vi "Unbox.vi"(10 "CustomeData in":refnum<class "CustomeData.lvclass">) -> (2 "data":i32)   [LabVIEW 2010, in "CustomeData.lvclass"]
uses:
  CustomeData.lvclass
  CustomeData.lvclass/CustomeData.ctl
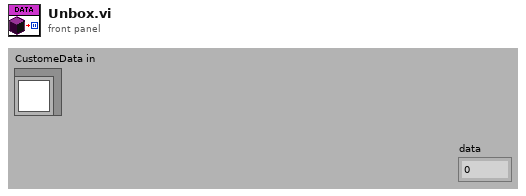
[diagram p1: front panel]
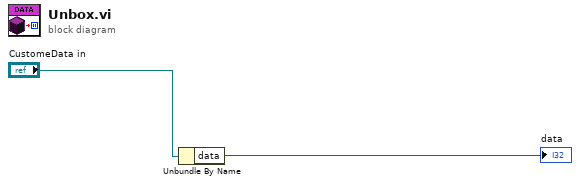
[diagram p0: block diagram]
diagram:
  n1 = Unbundle By Name("CustomeData in") -> ("data"=→"data":i32)
